vi "open kml.vi"() -> (1 "Open KML":string="<?xml version=\"1.0\" encoding=\"UTF-8\"?>\n<kml xmlns=\"http://www.opengis.net/kml/2.2\">")   [LabVIEW 2015, in "Biblioteka moduł map v3.lvlib" / "KML.lvlib"]
uses:
  KML.lvlib
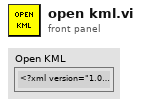
[diagram p1: front panel]
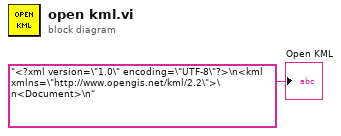
[diagram p0: block diagram]
diagram:
  "Open KML" <- "<?xml version=\"1.0\" encoding=\"UTF-8\"?>\n<kml xmlns=\"http://www.opengis.net/kml/2.2\">\n<Document>\n"
